vi "AlGaInPAs_v22.vi"(2 "Debug Mode":bool, 3 "Elapsed Time(s)":dbl, 4 "State":enum16{"Edit", "Start", "Run", "End", "Idle"}(ring), 5 "Argument List In":string[](array[string])) -> (0 "Status Out":string, 1 "Argument List Out":string[](array[string]))   [LabVIEW 2011]
uses:
  high_level_proc/source_dilution.ctl
  high_level_proc/source_noDilution.ctl
panel:
  in  "Ring":u16(ring)
  out "source array":refnum<vi>[](array[refnum])
  in  "Zn_bubbler":T1={"Dilution"=FALSE, "Calculated"=0, "MFC1 flow"=0.0, "MFC2 flow"=10.0, "MFC3 flow"=100.0, "Main"={"Flow"=0.0, "Prep"=FALSE, "Run"=FALSE, "Active"=FALSE, "Name"="Zn"}} caption="Al" {"Main"."Flow" format="%.2f"; "MFC1 flow" format="%.4f"; "MFC3 flow" format="%.1f"; "MFC2 flow" format="%.2f"; "Calculated" items=["Flow", "MFC1", "MFC2", "MFC3"]}
  in  "Al_bubbler":T2={"Flow"=0.0, "Prep"=FALSE, "Run"=FALSE, "Active"=FALSE, "Name"="Al"} caption="Al" {"Flow" format="%.2f"}
  in  "Se_bubbler":T1={"Dilution"=FALSE, "Calculated"=0, "MFC1 flow"=0.0, "MFC2 flow"=10.0, "MFC3 flow"=100.0, "Main"={"Flow"=0.0, "Prep"=FALSE, "Run"=FALSE, "Active"=FALSE, "Name"="Se"}} caption="Al" {"Main"."Flow" format="%.2f"; "MFC1 flow" format="%.4f"; "MFC3 flow" format="%.1f"; "MFC2 flow" format="%.2f"; "Calculated" items=["Flow", "MFC1", "MFC2", "MFC3"]}
  in  "P_bubbler":T2={"Flow"=0.0, "Prep"=FALSE, "Run"=FALSE, "Active"=FALSE, "Name"="P liq"} caption="Al" {"Flow" format="%.2f"}
  in  "As_gas":T2={"Flow"=0.0, "Prep"=FALSE, "Run"=FALSE, "Active"=FALSE, "Name"="As gas"} caption="Al" {"Flow" format="%.2f"}
  in  "P_gas":T2={"Flow"=0.0, "Prep"=FALSE, "Run"=FALSE, "Active"=FALSE, "Name"="P gas"} caption="Al" {"Flow" format="%.2f"}
  in  "In_bubbler":T2={"Flow"=0.0, "Prep"=FALSE, "Run"=FALSE, "Active"=FALSE, "Name"="In"} caption="Al" {"Flow" format="%.2f"}
  in  "Ga_bubbler":T1={"Dilution"=FALSE, "Calculated"=0, "MFC1 flow"=0.0, "MFC2 flow"=10.0, "MFC3 flow"=100.0, "Main"={"Flow"=0.0, "Prep"=FALSE, "Run"=FALSE, "Active"=FALSE, "Name"="Ga"}} caption="Al" {"Main"."Flow" format="%.2f"; "MFC1 flow" format="%.4f"; "MFC3 flow" format="%.1f"; "MFC2 flow" format="%.2f"; "Calculated" items=["Flow", "MFC1", "MFC2", "MFC3"]}
  out "prep_done":bool
  out "run started":bool
  out "first":bool=TRUE
  out "is OK?":bool
  in  "prep_time":dbl
  in  "Cancel":bool
  in  "OK":bool
  # "s"
  # "Add pre-run time to run time in editor."
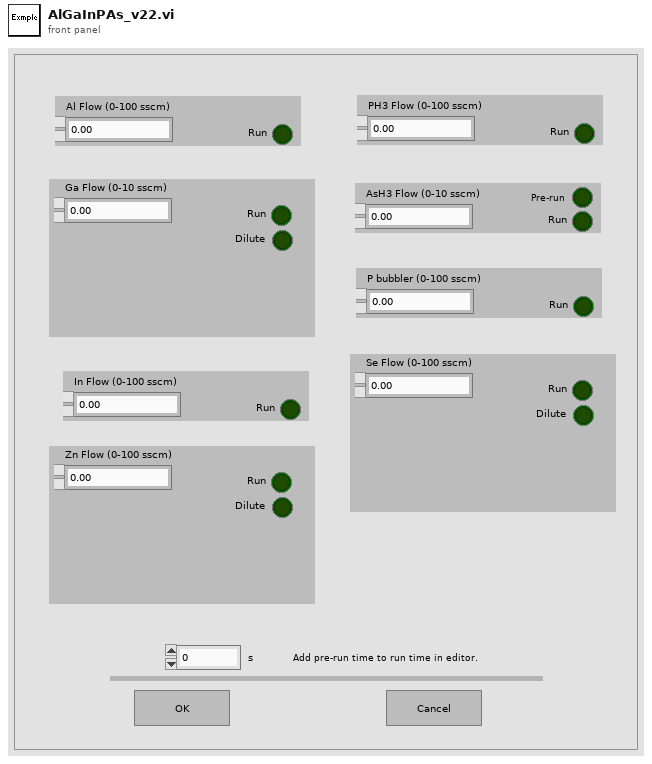
[diagram p1: front panel]
types:
  T1 = typedef "source_dilution.ctl" = cluster{"Dilution":bool, "Calculated":u16, "MFC1 flow":dbl, "MFC2 flow":dbl, "MFC3 flow":dbl, "Main":T2}
  T2 = typedef "source_noDilution.ctl" = cluster{"Flow":dbl, "Prep":bool, "Run":bool, "Active":bool, "Name":string}
  T3 = enum32{"Invalid", "Default", "Floating", "Floating/Auto-Hide", "Modal"}
  T4 = enum16{"Discrete", "Continuous", "Instantaneous", "Finite"}
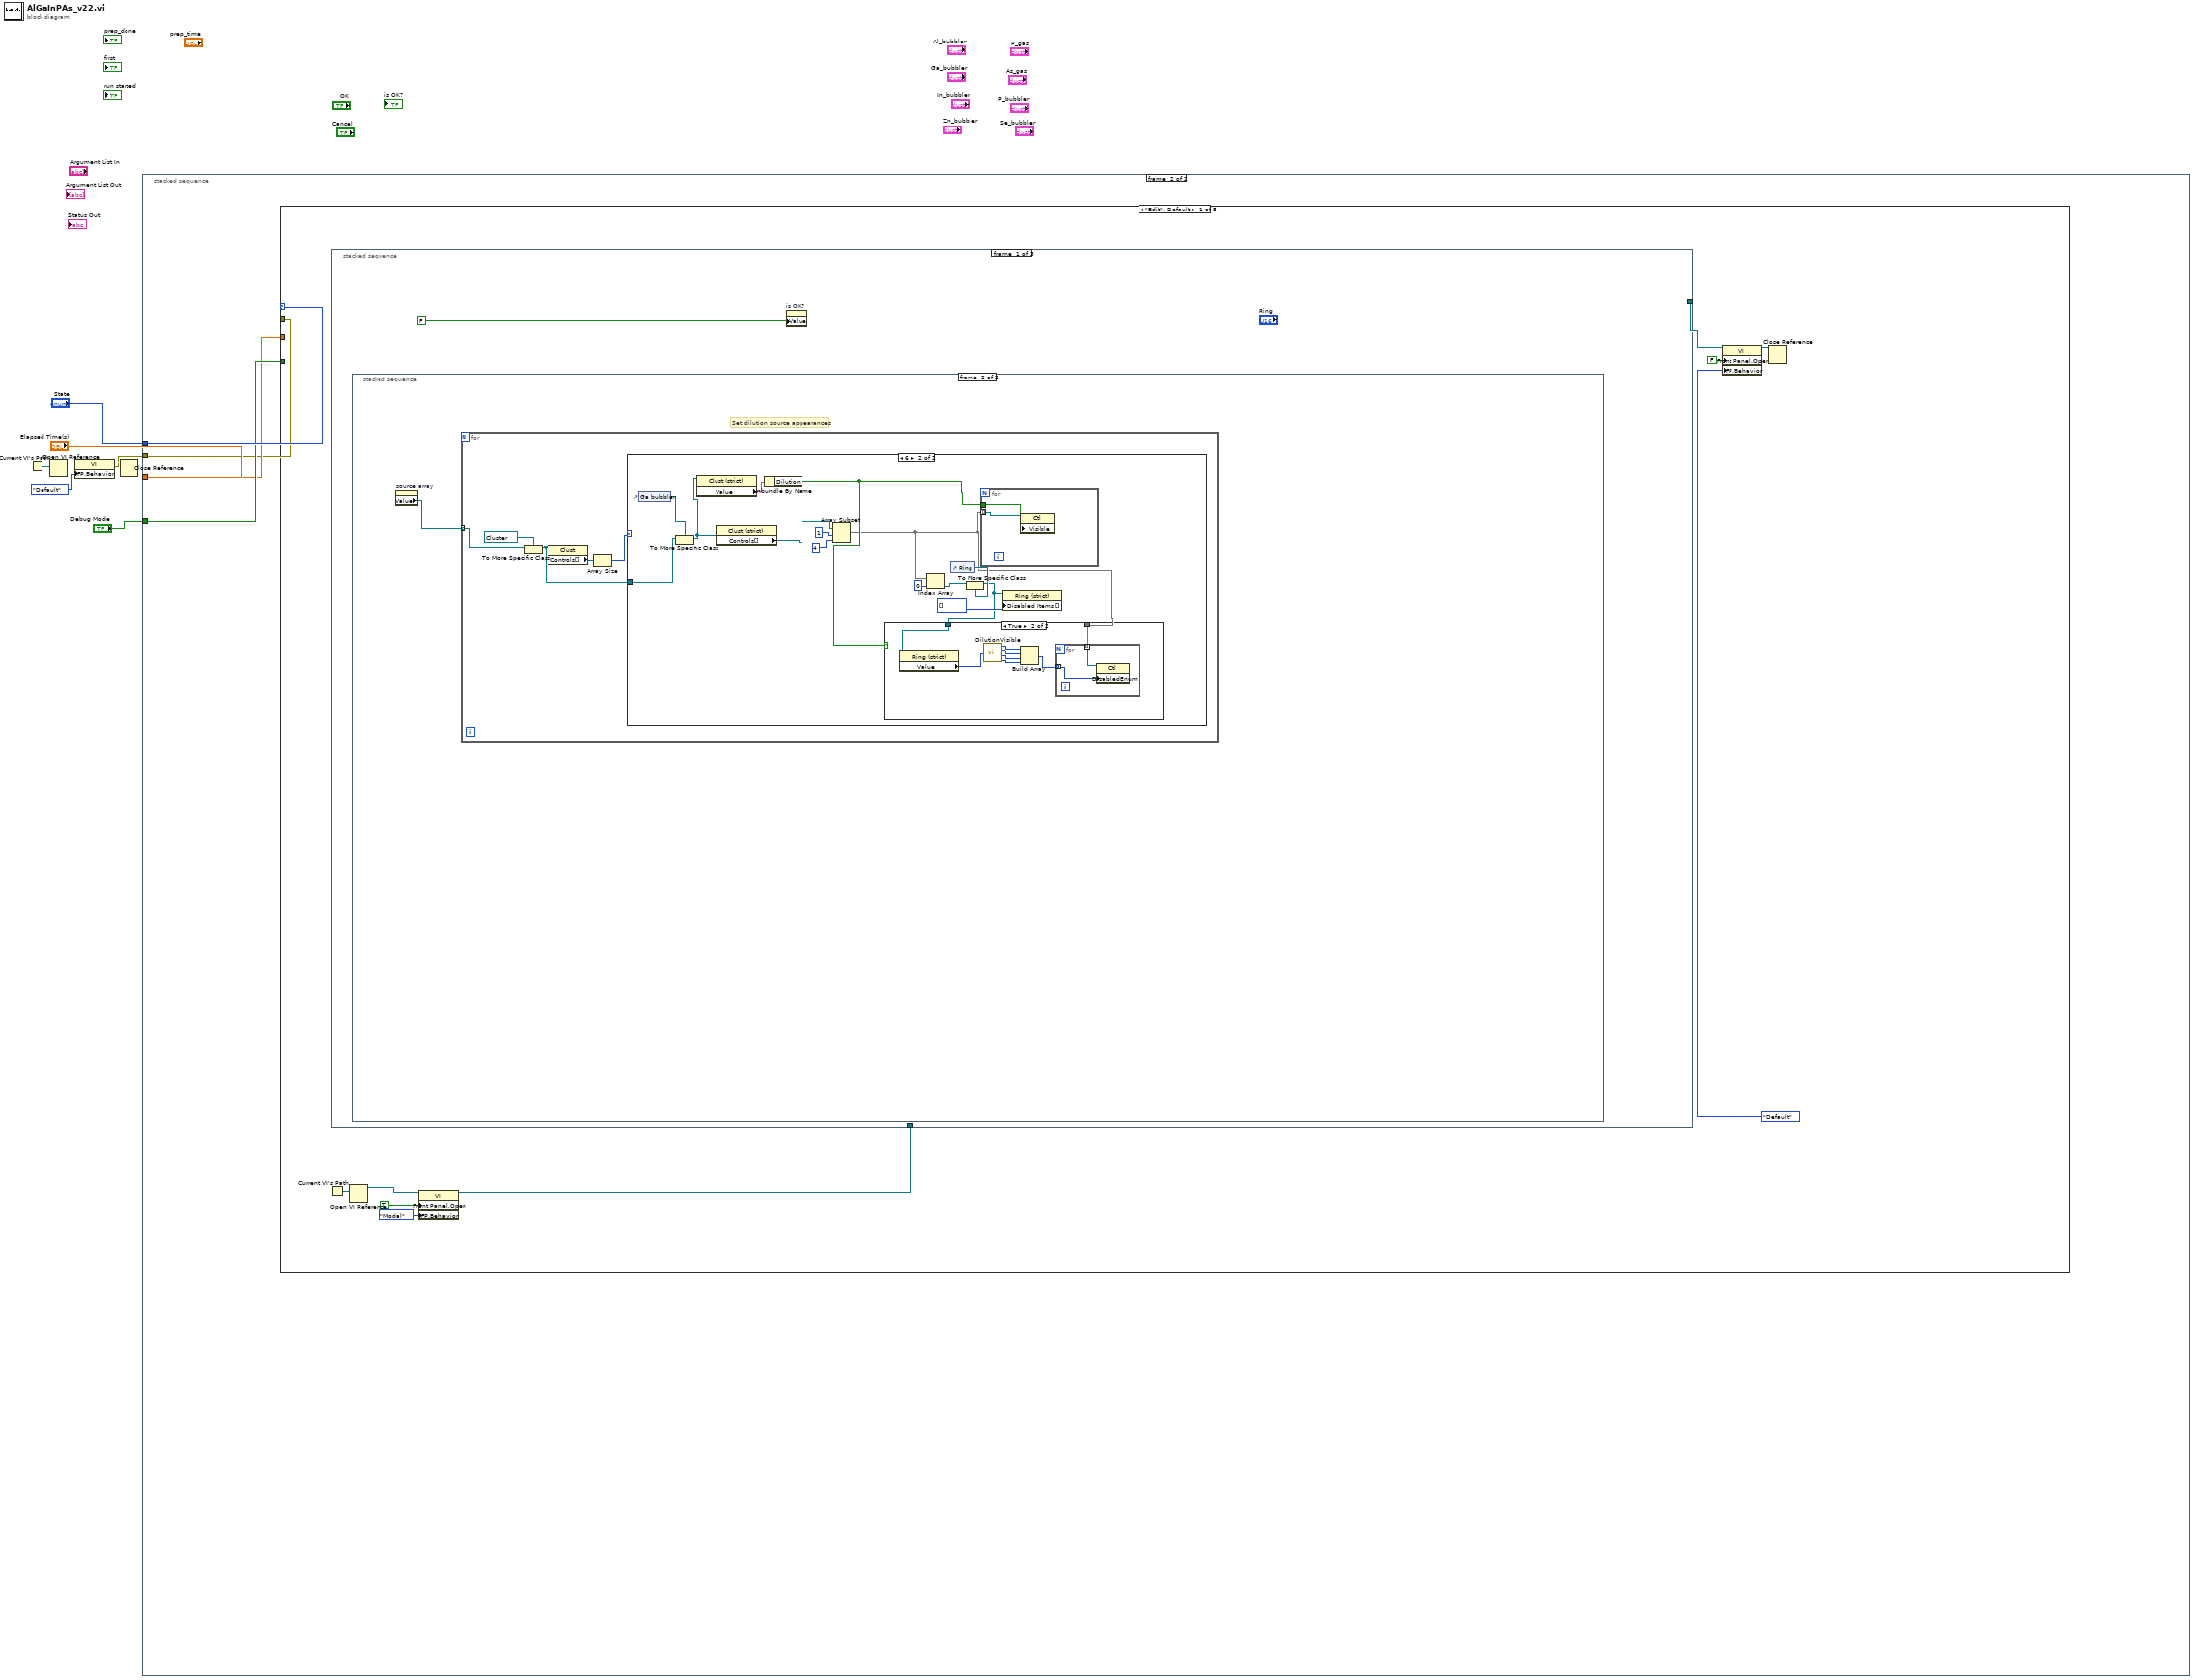
[diagram p0: block diagram]
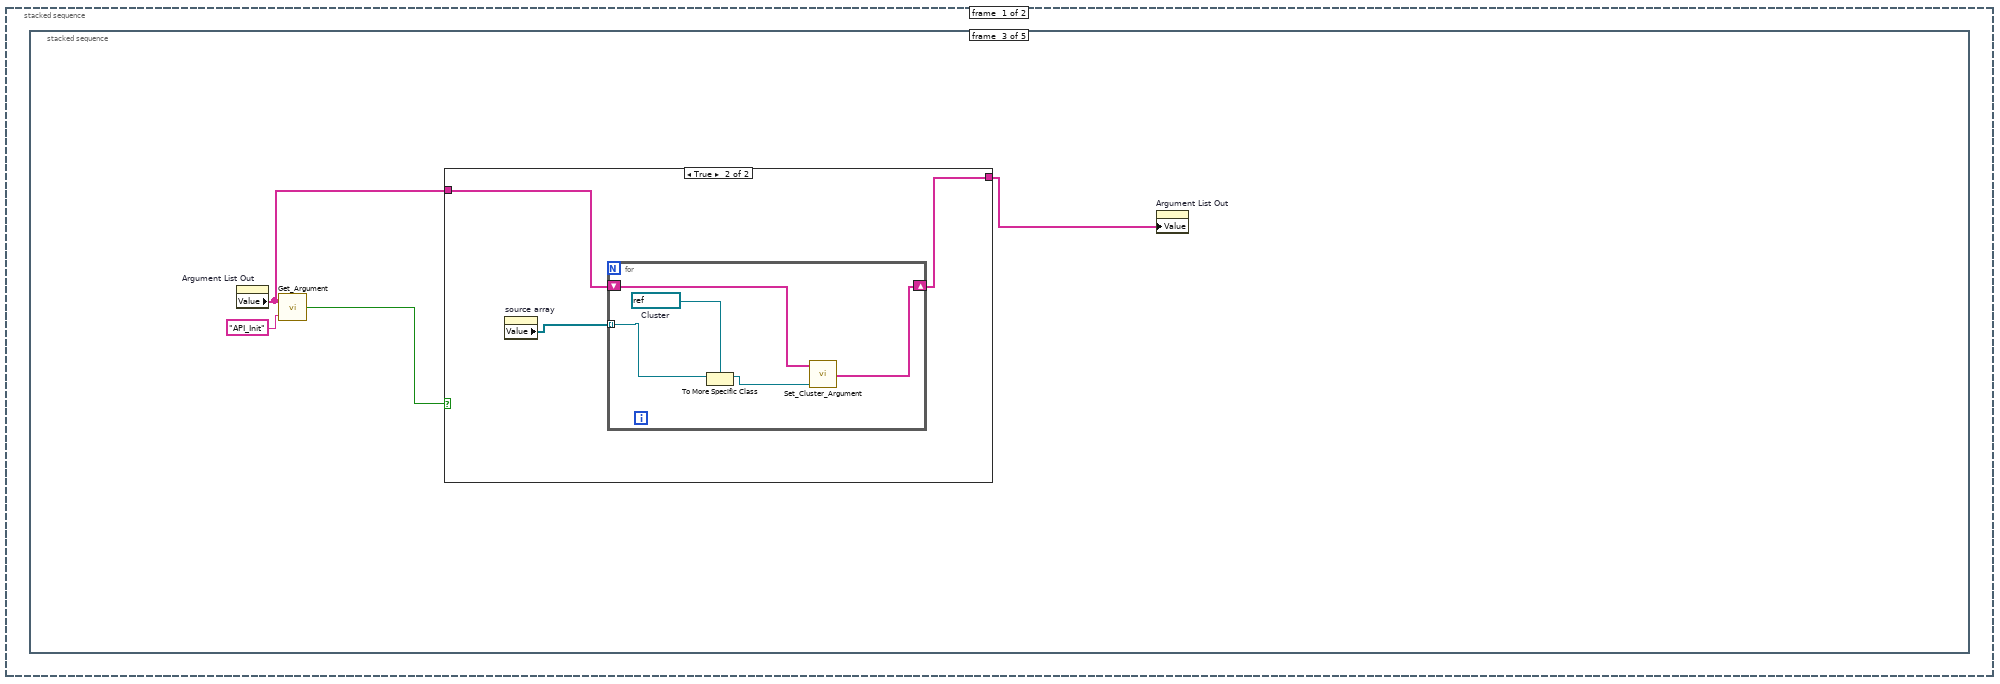
[diagram p2: hidden frame]
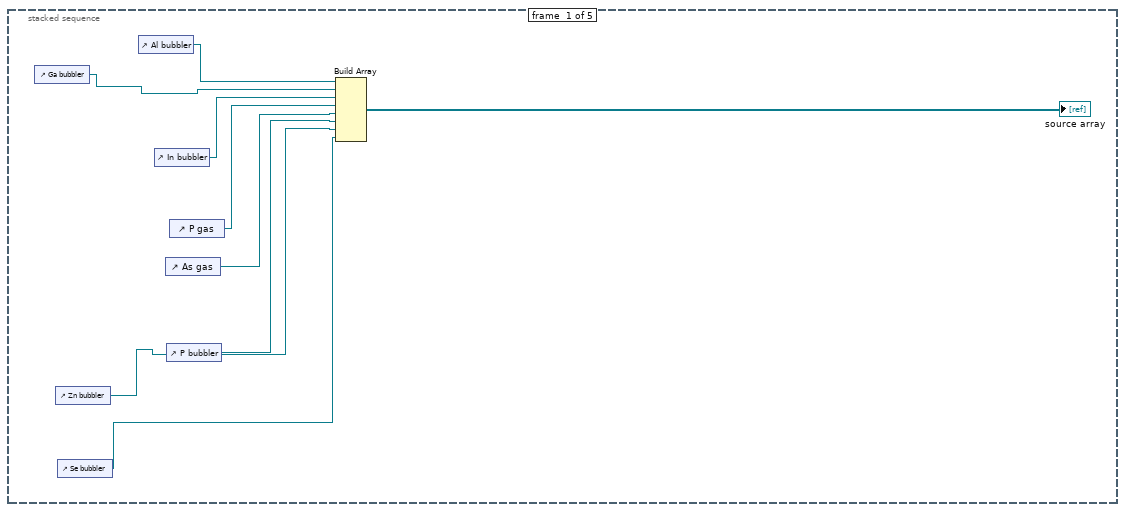
[diagram p3: hidden frame]
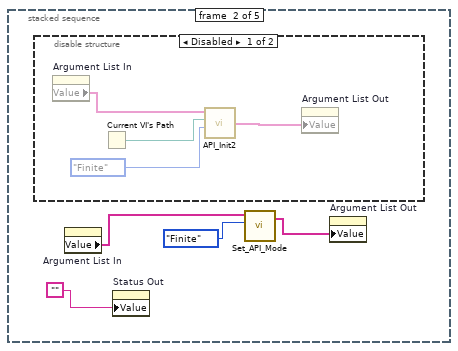
[diagram p4: hidden frame]
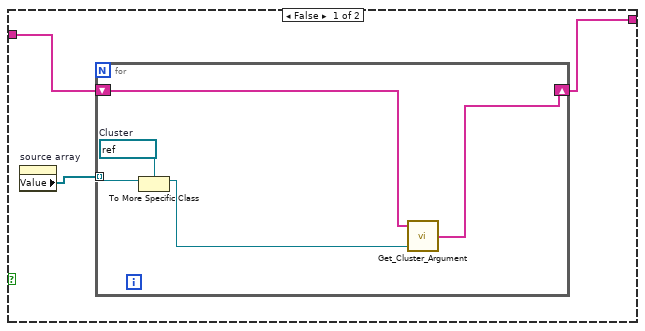
[diagram p6: hidden frame]
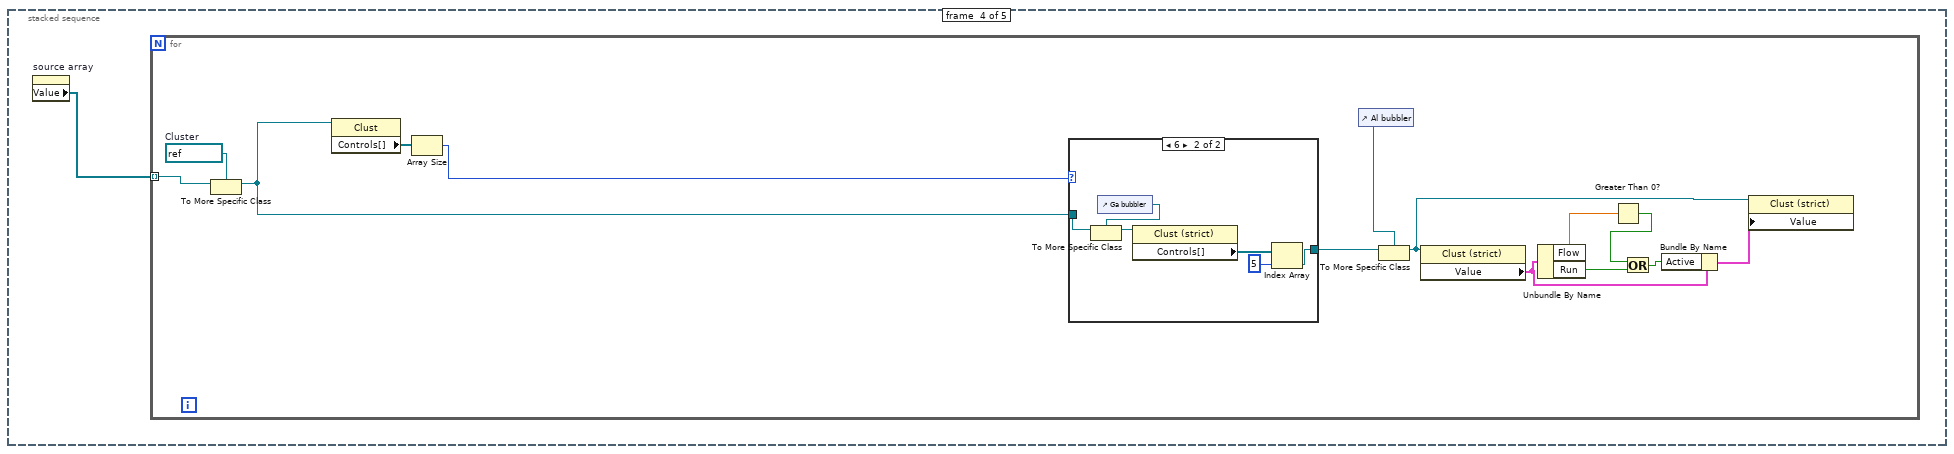
[diagram p7: hidden frame]
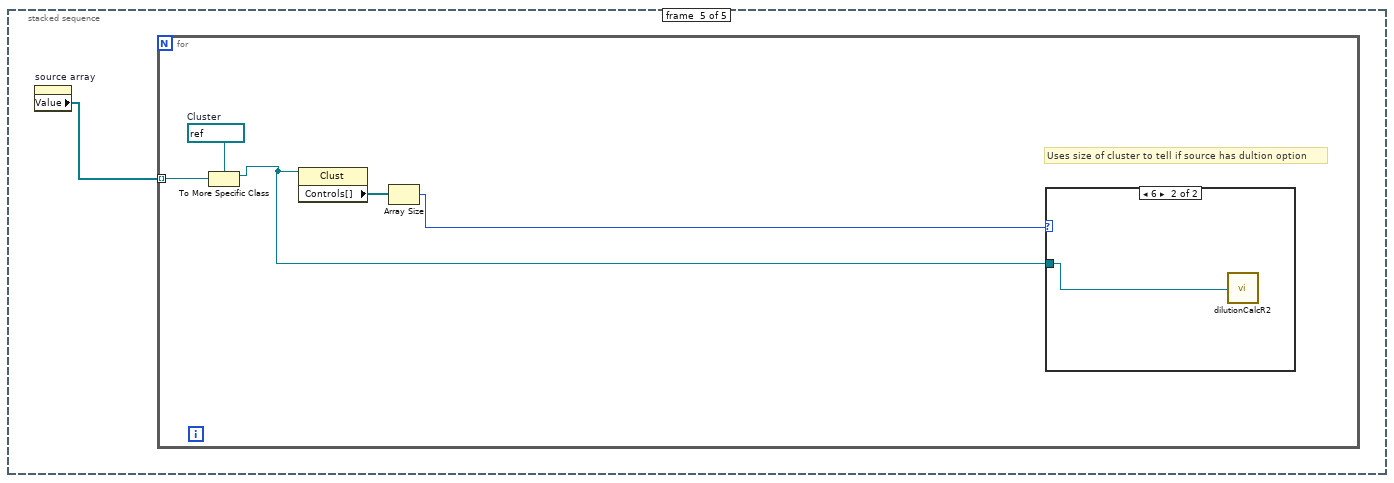
[diagram p9: hidden frame]
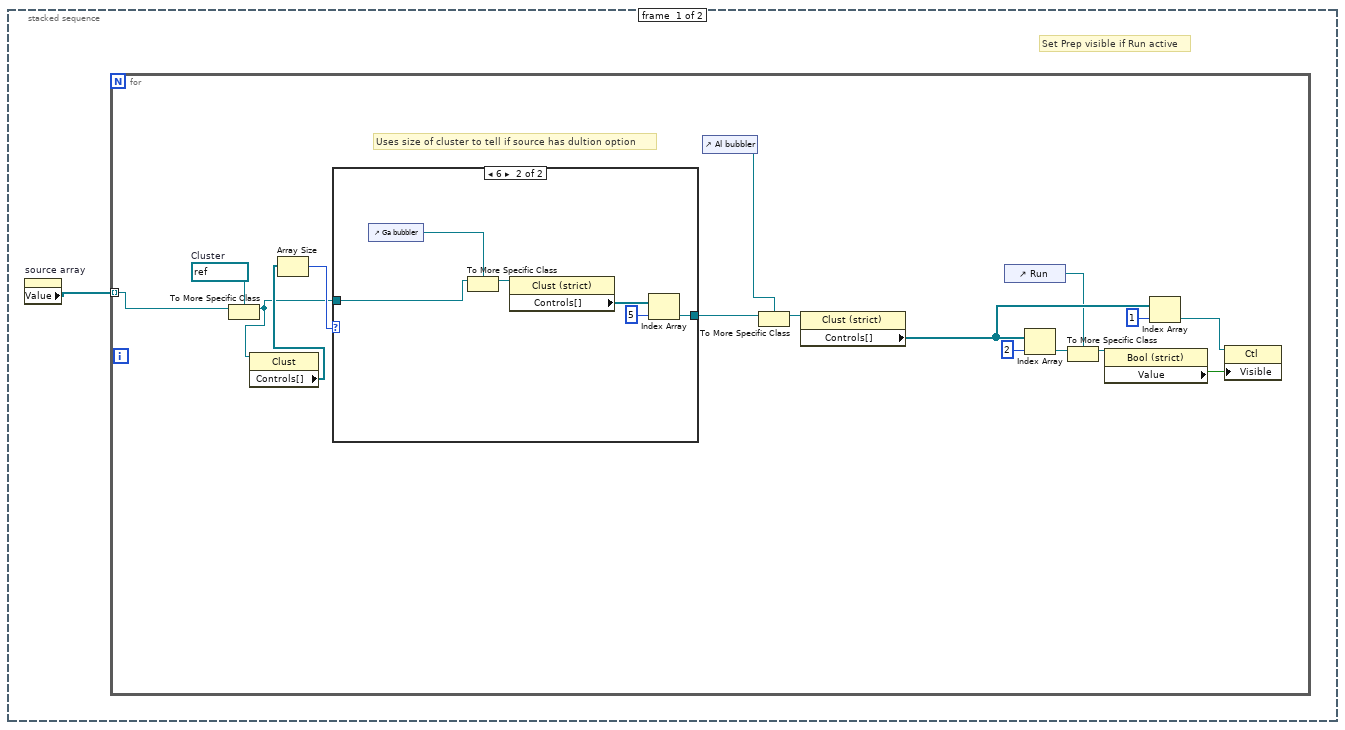
[diagram p11: hidden frame]
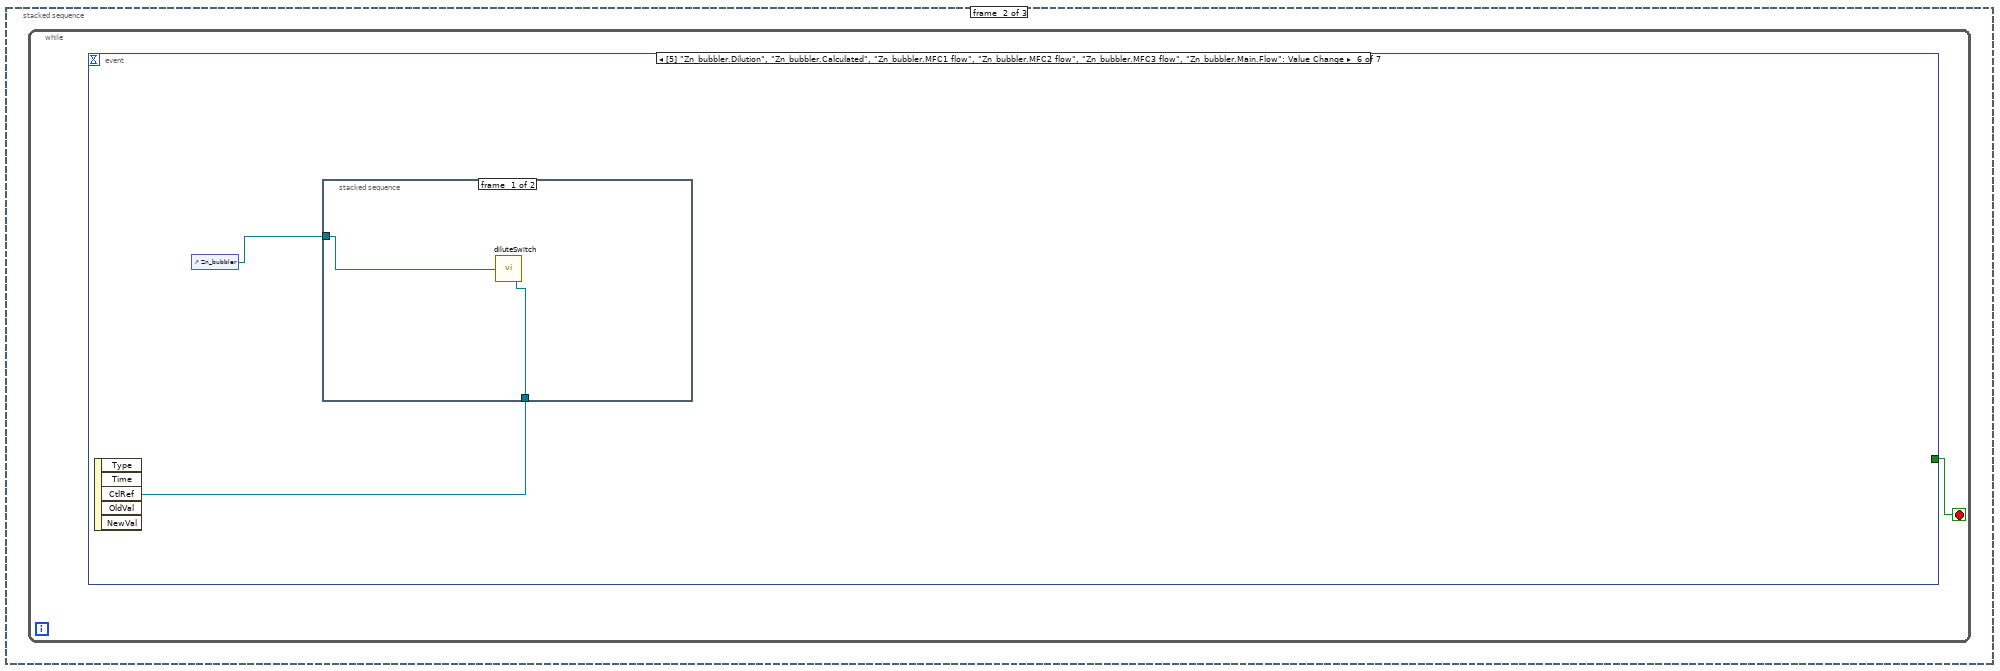
[diagram p15: hidden frame]
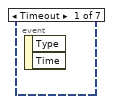
[diagram p16: hidden frame]
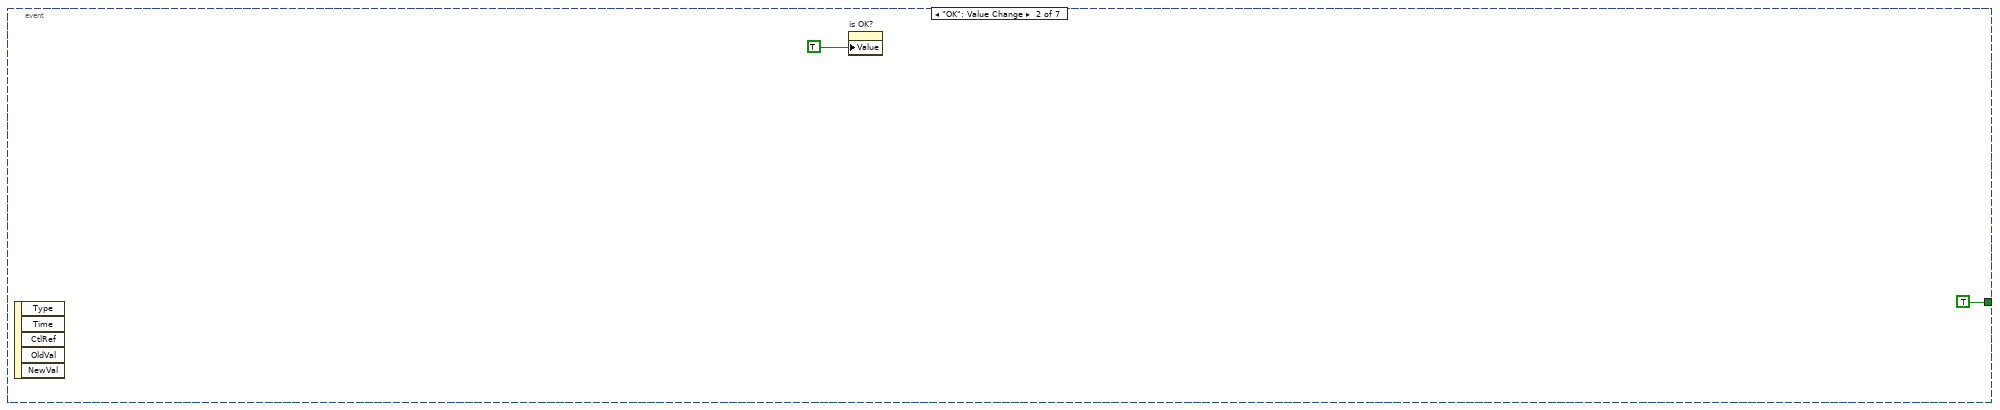
[diagram p17: hidden frame]
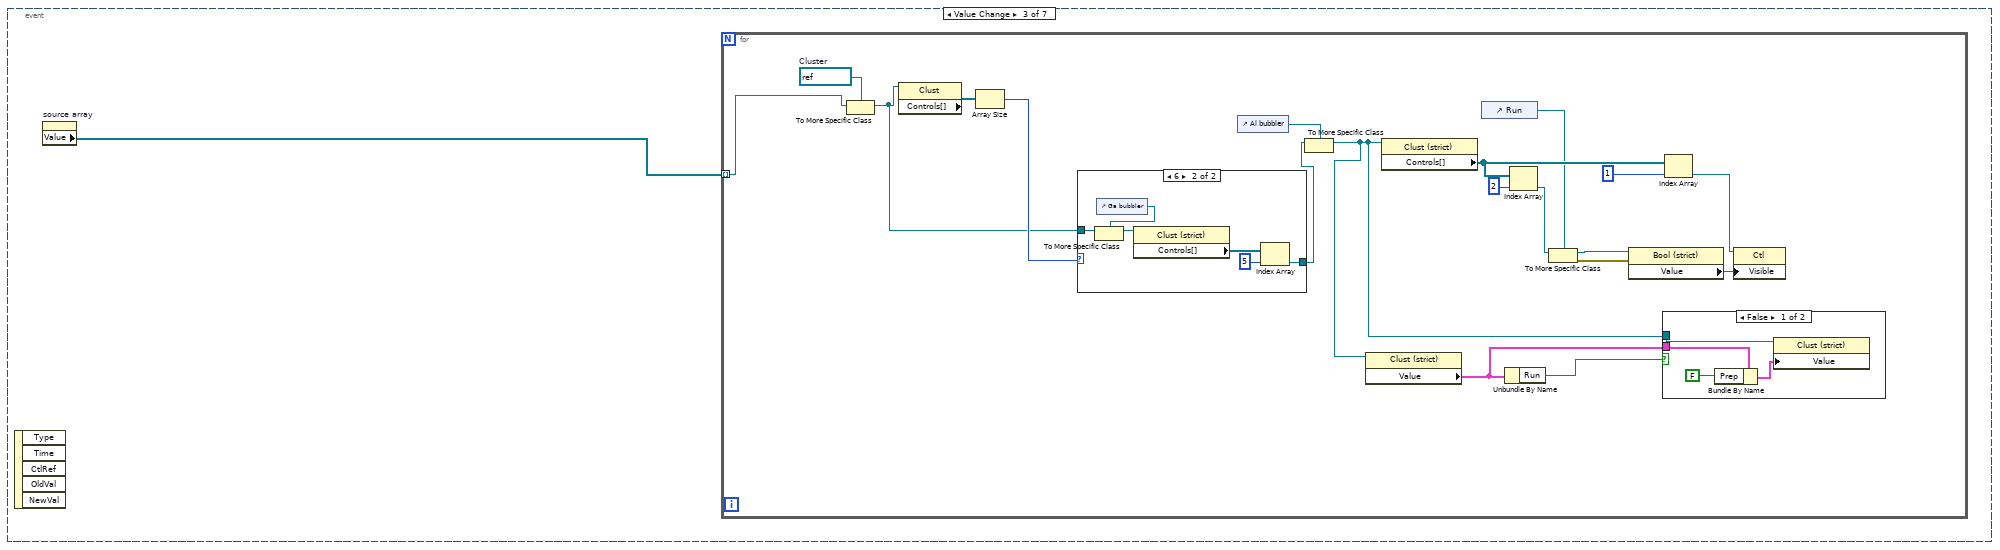
[diagram p18: hidden frame]
diagram:
  n1 = Current VI's Path() -> (path=w5:path)
  n2 = Open VI Reference(vi path=w5) -> (vi reference=w4:refnum<vi>)  [unwired: 1 in, 5 out]
  n3 = property class="VI"(reference=w4, "FP.Behavior"=T3."Default" ("Front Panel Window:Behavior")) -> (reference out=w2:refnum<vi>, error out=w1:errorcluster)  [unwired: 1 in]
  n4 = Close Reference(reference=w2) -> ()  [unwired: 1 in, 1 out]
  n5 = stacked-sequence {
    tunnel: "State" -> [_ w78]
    tunnel: "Debug Mode" -> [_ w77]
    tunnel: "Elapsed Time(s)" -> [_ w76]
    tunnel: w1 -> [_ w75]
    frame #0 {
      n6 = stacked-sequence {
        frame #0 {
          n7 = control-ref of="Ga bubbler"() -> (w12:refnum<vi>)
          n8 = control-ref of="Zn bubbler"() -> (w11:refnum<vi>)
          n9 = control-ref of="Se bubbler"() -> (w10:refnum<vi>)
          n10 = control-ref of="Al bubbler"() -> (w17:refnum<vi>)
          n11 = control-ref of="In bubbler"() -> (w16:refnum<vi>)
          n12 = control-ref of="As gas"() -> (w14:refnum<vi>)
          n13 = control-ref of="P bubbler"() -> (w13:refnum<vi>)
          n14 = control-ref of="P gas"() -> (w15:refnum<vi>)
          n15 = Build Array(w17, w12, w16, w15, w14, w13, w11, w10) -> (→"source array":refnum<vi>[])
        }
        frame #1 {
          n16 = disable-structure shown="Disabled" {
            frame Disabled {
              n17 = property on="Argument List In" class="Arr (strict)"() -> ("Value"=w25:string[])  [unwired: 2 in, 2 out]
              n18 = Current VI's Path() -> (path=w22:path)
              n19 = call "API_Init2.vi"("API Mode"=T4."Finite", "VI Path"=w22, "Argument List In"=w25) -> ("Argument List Out"=w24:string[])  [unwired: 1 in]
              n20 = property on="Argument List Out" class="Arr (strict)"("Value"=w24) -> ()  [unwired: 2 in, 2 out]
            }
            frame Enabled {
            }
          }
          n21 = property on="Argument List In" class="Arr (strict)"() -> ("Value"=w20:string[])  [unwired: 2 in, 2 out]
          n22 = property on="Status Out" class="Str"("Value"="") -> ()  [unwired: 2 in, 2 out]
          n23 = call "Set_API_Mode.vi"("API Mode"=T4."Finite", "Argument List In"=w20) -> ("Argument List Out"=w18:string[])  [unwired: 3 in]
          n24 = property on="Argument List Out" class="Arr (strict)"("Value"=w18) -> ()  [unwired: 2 in, 2 out]
        }
        frame #2 {
          n25 = property on="Argument List Out" class="Arr (strict)"() -> ("Value"=w27:string[])  [unwired: 2 in, 2 out]
          n26 = call "Get_Argument.vi"("Argument"="API_Init", "Argument List"=w27) -> ("Enabled"=w28:bool)
          n27 = case shown="True" w28 {
            tunnel: w27 -> [w32 w40]
            tunnel: [w30 w39] -> w26
            frame False {
              n28 = property on="source array" class="Arr (strict)"() -> ("Value"=w31:refnum<vi>[])  [unwired: 2 in, 2 out]
              n29 = for {
                shift-right: [w36] -> w30
                shift-left: w32 -> [w37]
                tunnel: w31 -> [w35] mode=indexing
                w33 = refnum<vi> refnum  # Cluster
                n30 = To More Specific Class(target class=w33, reference=w35) -> (specific class reference=w34:refnum<vi>)  [unwired: 1 in, 1 out]
                n31 = call "Get_Cluster_Argument.vi"("source"=w34, "Argument List In"=w37) -> ("Argument List Out"=w36:string[])  [unwired: 1 in]
              }
            }
            frame True {
              n32 = property on="source array" class="Arr (strict)"() -> ("Value"=w38:refnum<vi>[])  [unwired: 2 in, 2 out]
              n33 = for {
                shift-right: [w44] -> w39
                shift-left: w40 -> [w45]
                tunnel: w38 -> [w43] mode=indexing
                w42 = refnum<vi> refnum  # Cluster
                n34 = To More Specific Class(target class=w42, reference=w43) -> (specific class reference=w41:refnum<vi>)  [unwired: 1 in, 1 out]
                n35 = call "Set_Cluster_Argument.vi"("Clust Refnum"=w41, "Argument List In"=w45) -> ("Argument List Out"=w44:string[])  [unwired: 1 in]
              }
            }
          }
          n36 = property on="Argument List Out" class="Arr (strict)"("Value"=w26) -> ()  [unwired: 2 in, 2 out]
        }
        frame #3 {
          n37 = property on="source array" class="Arr (strict)"() -> ("Value"=w46:refnum<vi>[])  [unwired: 2 in, 2 out]
          n38 = for {
            tunnel: w46 -> [w49] mode=indexing
            w47 = refnum<vi> refnum  # Cluster
            n39 = To More Specific Class(target class=w47, reference=w49) -> (specific class reference=w48:refnum<vi>)  [unwired: 1 in, 1 out]
            n40 = property class="Clust"(reference=w48) -> ("Controls[]"=w51:refnum<vi>[])  [unwired: 1 in, 2 out]
            n41 = Array Size(array=w51) -> (size(s)=w52:i32)
            n42 = case shown="6" w52 {
              tunnel: [w61 w63] -> w50
              tunnel: w48 -> [w61 w66]
              frame Default {
              }
              frame 6 {
                n43 = control-ref of="Ga bubbler"() -> (w62:refnum<vi>)
                n44 = To More Specific Class(target class=w62, reference=w66) -> (specific class reference=w65:refnum<vi>)  [unwired: 1 in, 1 out]
                n45 = property class="Clust (strict)"(reference=w65) -> ("Controls[]"=w64:refnum<vi>[])  [unwired: 1 in, 2 out]
                n46 = Index Array(array=w64, index=5) -> (element=w63:refnum<vi>)
              }
            }
            n47 = control-ref of="Al bubbler"() -> (w54:refnum<vi>)
            n48 = To More Specific Class(target class=w54, reference=w50) -> (specific class reference=w53:refnum<vi>)  [unwired: 1 in, 1 out]
            n49 = property class="Clust (strict)"(reference=w53) -> ("Value"=w57:T2)  [unwired: 1 in, 2 out]
            n50 = Unbundle By Name(w57) -> ("Flow"=w60:dbl, "Run"=w58:bool)
            n51 = Greater Than 0?(x=w60) -> (x > 0?=w59:bool)
            n52 = Or(x=w59, y=w58) -> (x .or. y?=w55:bool)
            n53 = Bundle By Name(cluster=w57, "Active"=w55) -> (w56:T2)
            n54 = property class="Clust (strict)"(reference=w53, "Value"=w56) -> ()  [unwired: 1 in, 2 out]
          }
        }
        frame #4 {
          n55 = property on="source array" class="Arr (strict)"() -> ("Value"=w68:refnum<vi>[])  [unwired: 2 in, 2 out]
          n56 = for {
            tunnel: w68 -> [w72] mode=indexing
            w70 = refnum<vi> refnum  # Cluster
            # "Uses size of cluster to tell if source has dultion option"
            n57 = To More Specific Class(target class=w70, reference=w72) -> (specific class reference=w71:refnum<vi>)  [unwired: 1 in, 1 out]
            n58 = property class="Clust"(reference=w71) -> ("Controls[]"=w69:refnum<vi>[])  [unwired: 1 in, 2 out]
            n59 = Array Size(array=w69) -> (size(s)=w73:i32)
            n60 = case shown="6" w73 {
              tunnel: w71 -> [_ w74]
              frame Default {
              }
              frame 6 {
                n61 = call "dilutionCalcR2.vi"("Clust Refnum"=w74) -> ()
              }
            }
          }
        }
      }
    }
    frame #1 {
      n62 = case shown="\"Edit\", Default" w78 {
        tunnel: w77 -> [_ w214 w230 _ _]
        tunnel: w76 -> [_ _ w231 _ _]
        tunnel: w75 -> [_ _ _ _ _]
        frame "Edit", Default {
          n63 = Current VI's Path() -> (path=w83:path)
          n64 = Open VI Reference(vi path=w83) -> (vi reference=w82:refnum<vi>)  [unwired: 1 in, 5 out]
          n65 = property class="VI"(reference=w82, "Front Panel.Open"=TRUE ("Front Panel Window:Open"), "FP.Behavior"=T3."Modal" ("Front Panel Window:Behavior")) -> (reference out=w80:refnum<vi>)  [unwired: 1 in, 1 out]
          n66 = stacked-sequence {
            tunnel: [_ _ w197] -> w85
            tunnel: w80 -> [_ _ w197]
            frame #0 {
              n67 = stacked-sequence {
                frame #0 {
                  # "Set Prep visible if Run active"
                  n68 = property on="source array" class="Arr (strict)"() -> ("Value"=w89:refnum<vi>[])  [unwired: 2 in, 2 out]
                  n69 = for {
                    tunnel: w89 -> [w94] mode=indexing
                    w93 = refnum<vi> refnum  # Cluster
                    # "Uses size of cluster to tell if source has dultion option"
                    n70 = To More Specific Class(target class=w93, reference=w94) -> (specific class reference=w90:refnum<vi>)  [unwired: 1 in, 1 out]
                    n71 = property class="Clust"(reference=w90) -> ("Controls[]"=w92:refnum<vi>[])  [unwired: 1 in, 2 out]
                    n72 = Array Size(array=w92) -> (size(s)=w91:i32)
                    n73 = case shown="6" w91 {
                      tunnel: w90 -> [w106 w109]
                      tunnel: [w106 w110] -> w96
                      frame Default {
                      }
                      frame 6 {
                        n74 = control-ref of="Ga bubbler"() -> (w107:refnum<vi>)
                        n75 = To More Specific Class(target class=w107, reference=w109) -> (specific class reference=w108:refnum<vi>)  [unwired: 1 in, 1 out]
                        n76 = property class="Clust (strict)"(reference=w108) -> ("Controls[]"=w112:refnum<vi>[])  [unwired: 1 in, 2 out]
                        n77 = Index Array(array=w112, index=5) -> (element=w110:refnum<vi>)
                      }
                    }
                    n78 = control-ref of="Al bubbler"() -> (w97:refnum<vi>)
                    n79 = To More Specific Class(target class=w97, reference=w96) -> (specific class reference=w103:refnum<vi>)  [unwired: 1 in, 1 out]
                    n80 = property class="Clust (strict)"(reference=w103) -> ("Controls[]"=w102:refnum<vi>[])  [unwired: 1 in, 2 out]
                    n81 = control-ref of="Run"() -> (w95:refnum<vi>)
                    n82 = Index Array(array=w102, index=2) -> (element=w100:refnum<vi>)
                    n83 = To More Specific Class(target class=w95, reference=w100) -> (specific class reference=w99:refnum<vi>)  [unwired: 1 in, 1 out]
                    n84 = property class="Bool (strict)"(reference=w99) -> ("Value"=w98:bool)  [unwired: 1 in, 2 out]
                    n85 = Index Array(array=w102, index=1) -> (element=w104:refnum<vi>)
                    n86 = property class="Ctl"(reference=w104, "Visible"=w98) -> ()  [unwired: 1 in, 2 out]
                  }
                }
                frame #1 {
                  # "Set dilution source appearances"
                  n87 = property on="source array" class="Arr (strict)"() -> ("Value"=w113:refnum<vi>[])  [unwired: 2 in, 2 out]
                  n88 = for {
                    tunnel: w113 -> [w118] mode=indexing
                    n89 = To More Specific Class(target class=refnum<vi> refnum, reference=w118) -> (specific class reference=w114:refnum<vi>)  [unwired: 1 in, 1 out]
                    n90 = property class="Clust"(reference=w114) -> ("Controls[]"=w116:refnum<vi>[])  [unwired: 1 in, 2 out]
                    n91 = Array Size(array=w116) -> (size(s)=w115:i32)
                    n92 = case shown="6" w115 {
                      tunnel: w114 -> [_ w132]
                      frame Default {
                      }
                      frame 6 {
                        n93 = control-ref of="Ga bubbler"() -> (w131:refnum<vi>)
                        n94 = To More Specific Class(target class=w131, reference=w132) -> (specific class reference=w129:refnum<vi>)  [unwired: 1 in, 1 out]
                        n95 = property class="Clust (strict)"(reference=w129) -> ("Value"=w130:T1)  [unwired: 1 in, 2 out]
                        n96 = property class="Clust (strict)"(reference=w129) -> ("Controls[]"=w128:refnum<vi>[])  [unwired: 1 in, 2 out]
                        n97 = Unbundle By Name(w130) -> ("Dilution"=w122:bool)
                        n98 = Array Subset(array=w128, index=1, length=4) -> (w119:refnum<vi>[])
                        n99 = Index Array(array=w119, index=0) -> (element=w121:refnum<vi>)
                        n100 = control-ref of="Ring"() -> (w124:refnum<vi>)
                        n101 = To More Specific Class(target class=w124, reference=w121) -> (specific class reference=w120:refnum<vi>)  [unwired: 1 in, 1 out]
                        n102 = case shown="True" w122 {
                          tunnel: w120 -> [_ w140]
                          tunnel: w119 -> [_ w133]
                          frame False {
                          }
                          frame True {
                            n103 = property class="Ring (strict)"(reference=w140) -> ("Value"=w139:u16)  [unwired: 1 in, 2 out]
                            n104 = call "DilutionVisible.vi"("calculated"=w139) -> ("flow"=w138:u16, "MFC1"=w137:u16, "MFC2"=w136:u16, "MFC3"=w135:u16)
                            n105 = Build Array(w138, w137, w136, w135) -> (w134:u16[])
                            n106 = for {
                              tunnel: w134 -> [w141] mode=indexing
                              tunnel: w133 -> [w142] mode=indexing
                              n107 = property class="Ctl"(reference=w142, "DisabledEnum"=w141) -> ()  [unwired: 1 in, 2 out]
                            }
                          }
                        }
                        n108 = for {
                          tunnel: w119 -> [w144] mode=indexing
                          tunnel: w122 -> [w143]
                          n109 = property class="Ctl"(reference=w144, "Visible"=w143) -> ()  [unwired: 1 in, 2 out]
                        }
                        n110 = property class="Ring (strict)"(reference=w120, "Disabled Items []"=i32[] []) -> ()  [unwired: 1 in, 2 out]
                      }
                    }
                  }
                }
              }
              n111 = property on="is OK?" class="Bool (strict)"("Value"=FALSE ("is OK?")) -> ()  [unwired: 2 in, 2 out]
            }
            frame #1 {
              n112 = while {
                stop <- w145 stop-if-true
                n113 = event shown="[5] \"Zn_bubbler.Dilution\", \"Zn_bubbler.Calculated\", \"Zn_bubbler.MFC1 flow\", \"Zn_bubbler.MFC2 flow\", \"Zn_bubbler.MFC3 flow\", \"Zn_bubbler.Main.Flow\": Value Change" {
                  selector: _ -> [_ _ _ _ _ _ _]
                  dyn-events: _ -> [_ _ _ _ _ _ _]
                  timeout: _ -> [_ _ _ _ _ _ _]
                  tunnel: [_ TRUE _ TRUE _ _ _] -> w145
                  event Timeout {
                    n114 = event-data() -> ()  [unwired: 1 in, 2 out]
                  }
                  event "OK": Value Change {
                    n115 = event-data() -> ()  [unwired: 1 in, 5 out]
                    n116 = property on="is OK?" class="Bool (strict)"("Value"=TRUE ("is OK?")) -> ()  [unwired: 2 in, 2 out]
                  }
                  event Value Change {
                    n117 = event-data() -> ()  [unwired: 1 in, 5 out]
                    n118 = property on="source array" class="Arr (strict)"() -> ("Value"=w148:refnum<vi>[])  [unwired: 2 in, 2 out]
                    n119 = for {
                      tunnel: w148 -> [w151] mode=indexing
                      w149 = refnum<vi> refnum  # Cluster
                      n120 = To More Specific Class(target class=w149, reference=w151) -> (specific class reference=w150:refnum<vi>)  [unwired: 1 in, 1 out]
                      n121 = property class="Clust"(reference=w150) -> ("Controls[]"=w153:refnum<vi>[])  [unwired: 1 in, 2 out]
                      n122 = Array Size(array=w153) -> (size(s)=w152:i32)
                      n123 = case shown="6" w152 {
                        tunnel: w150 -> [w168 w171]
                        tunnel: [w168 w172] -> w155
                        frame Default {
                        }
                        frame 6 {
                          n124 = control-ref of="Ga bubbler"() -> (w169:refnum<vi>)
                          n125 = To More Specific Class(target class=w169, reference=w171) -> (specific class reference=w170:refnum<vi>)  [unwired: 1 in, 1 out]
                          n126 = property class="Clust (strict)"(reference=w170) -> ("Controls[]"=w174:refnum<vi>[])  [unwired: 1 in, 2 out]
                          n127 = Index Array(array=w174, index=5) -> (element=w172:refnum<vi>)
                        }
                      }
                      n128 = control-ref of="Al bubbler"() -> (w159:refnum<vi>)
                      n129 = To More Specific Class(target class=w159, reference=w155) -> (specific class reference=w156:refnum<vi>)  [unwired: 1 in, 1 out]
                      n130 = property class="Clust (strict)"(reference=w156) -> ("Value"=w158:T2)  [unwired: 1 in, 2 out]
                      n131 = property class="Clust (strict)"(reference=w156) -> ("Controls[]"=w165:refnum<vi>[])  [unwired: 1 in, 2 out]
                      n132 = control-ref of="Run"() -> (w154:refnum<vi>)
                      n133 = Unbundle By Name(w158) -> ("Run"=w157:bool)
                      n134 = Index Array(array=w165, index=2) -> (element=w163:refnum<vi>)
                      n135 = To More Specific Class(target class=w154, reference=w163) -> (specific class reference=w162:refnum<vi>, error out=w161:errorcluster)  [unwired: 1 in]
                      n136 = property class="Bool (strict)"(reference=w162, error in=w161) -> ("Value"=w160:bool)  [unwired: 2 out]
                      n137 = case shown="False" w157 {
                        tunnel: w158 -> [w178 _]
                        tunnel: w156 -> [w175 _]
                        frame False {
                          n138 = Bundle By Name(cluster=w178, "Prep"=FALSE) -> (w176:T2)
                          n139 = property class="Clust (strict)"(reference=w175, "Value"=w176) -> ()  [unwired: 1 in, 2 out]
                        }
                        frame True {
                        }
                      }
                      n140 = Index Array(array=w165, index=1) -> (element=w166:refnum<vi>)
                      n141 = property class="Ctl"(reference=w166, "Visible"=w160) -> ()  [unwired: 1 in, 2 out]
                    }
                  }
                  event "Cancel": Value Change {
                    n142 = event-data() -> ()  [unwired: 1 in, 5 out]
                  }
                  event Value Change {
                    n143 = event-data() -> ("CtlRef"=w180:refnum<vi>)  [unwired: 1 in, 4 out]
                    n144 = control-ref of="Ga_bubbler"() -> (w181:refnum<vi>)
                    n145 = stacked-sequence {
                      tunnel: w181 -> [w183 w184]
                      tunnel: w180 -> [w182 _]
                      frame #0 {
                        n146 = call "diluteSwitch.vi"("Ctl Refnum"=w182, "Clust Refnum"=w183) -> ()
                      }
                      frame #1 {
                        n147 = call "dilutionCalcR2.vi"("Clust Refnum"=w184) -> ()
                      }
                    }
                  }
                  event Value Change {
                    n148 = event-data() -> ("CtlRef"=w185:refnum<vi>)  [unwired: 1 in, 4 out]
                    n149 = control-ref of="Zn_bubbler"() -> (w186:refnum<vi>)
                    n150 = stacked-sequence {
                      tunnel: w186 -> [w188 w189]
                      tunnel: w185 -> [w187 _]
                      frame #0 {
                        n151 = call "diluteSwitch.vi"("Ctl Refnum"=w187, "Clust Refnum"=w188) -> ()
                      }
                      frame #1 {
                        n152 = call "dilutionCalcR2.vi"("Clust Refnum"=w189) -> ()
                      }
                    }
                  }
                  event Value Change {
                    n153 = event-data() -> ("CtlRef"=w190:refnum<vi>)  [unwired: 1 in, 4 out]
                    n154 = control-ref of="Se_bubbler"() -> (w191:refnum<vi>)
                    n155 = stacked-sequence {
                      tunnel: w191 -> [w193 w194]
                      tunnel: w190 -> [w192 _]
                      frame #0 {
                        n156 = call "diluteSwitch.vi"("Ctl Refnum"=w192, "Clust Refnum"=w193) -> ()
                      }
                      frame #1 {
                        n157 = call "dilutionCalcR2.vi"("Clust Refnum"=w194) -> ()
                      }
                    }
                  }
                }
              }
            }
            frame #2 {
              n158 = property on="Argument List Out" class="Arr (strict)"() -> ("Value"=w196:string[])  [unwired: 2 in, 2 out]
              n159 = property on="is OK?" class="Bool (strict)"() -> ("Value"=w198:bool)  [unwired: 2 in, 2 out]
              n160 = case shown="True" w198 {
                tunnel: w196 -> [w199 w205]
                tunnel: [w199 w201] -> w195
                frame False {
                }
                frame True {
                  n161 = property on="source array" class="Arr (strict)"() -> ("Value"=w204:refnum<vi>[])  [unwired: 2 in, 2 out]
                  n162 = for {
                    shift-right: [w209] -> w202
                    shift-left: w205 -> [w210]
                    tunnel: w204 -> [w208] mode=indexing
                    w207 = refnum<vi> refnum  # Cluster
                    n163 = To More Specific Class(target class=w207, reference=w208) -> (specific class reference=w206:refnum<vi>)  [unwired: 1 in, 1 out]
                    n164 = call "Set_Cluster_Argument.vi"("Clust Refnum"=w206, "Argument List In"=w210) -> ("Argument List Out"=w209:string[])  [unwired: 1 in]
                  }
                  n165 = call "Set_Argument.vi"("Enable"=FALSE, "Argument"="API_Init", "Argument List In"=w202) -> ("Argument List Out"=w201:string[])
                }
              }
              n166 = property on="Argument List Out" class="Arr (strict)"("Value"=w195) -> ()  [unwired: 2 in, 2 out]
            }
          }
          n167 = property class="VI"(reference=w85, "Front Panel.Open"=FALSE ("Front Panel Window:Open"), "FP.Behavior"=T3."Default" ("Front Panel Window:Behavior")) -> (reference out=w86:refnum<vi>)  [unwired: 1 in, 1 out]
          n168 = Close Reference(reference=w86) -> ()  [unwired: 1 in, 1 out]
        }
        frame "Start" {
          n169 = property on="prep_time" class="DigNum (strict)"() -> ("Value"=w217:dbl)  [unwired: 2 in, 2 out]
          n170 = Greater Than 0?(x=w217) -> (x > 0?=w216:bool)
          n171 = Not(x=w214) -> (.not. x?=w213:bool)
          n172 = property on="Argument List Out" class="Arr (strict)"() -> ("Value"=w212:string[])  [unwired: 2 in, 2 out]
          n173 = And(x=w213, y=w216) -> (x .and. y?=w215:bool)
          n174 = call "Set_Argument.vi"("Enable"=FALSE, "Argument"="run_started", "Argument List In"=w212) -> ("Argument List Out"=w211:string[])
          n175 = case shown="True" w215 {
            frame False {
            }
            frame True {
              n176 = property on="Ga_bubbler" class="Clust (strict)"() -> ("Value"=w226:T1)  [unwired: 2 in, 2 out]
              n177 = property on="Zn_bubbler" class="Clust (strict)"() -> ("Value"=w220:T1)  [unwired: 2 in, 2 out]
              n178 = property on="Al_bubbler" class="Clust (strict)"() -> ("Value"=w227:T2)  [unwired: 2 in, 2 out]
              n179 = property on="In_bubbler" class="Clust (strict)"() -> ("Value"=w225:T2)  [unwired: 2 in, 2 out]
              n180 = property on="P_gas" class="Clust (strict)"() -> ("Value"=w224:T2)  [unwired: 2 in, 2 out]
              n181 = property on="Se_bubbler" class="Clust (strict)"() -> ("Value"=w221:T1)  [unwired: 2 in, 2 out]
              n182 = property on="As_gas" class="Clust (strict)"() -> ("Value"=w223:T2)  [unwired: 2 in, 2 out]
              n183 = property on="P_bubbler" class="Clust (strict)"() -> ("Value"=w222:T2)  [unwired: 2 in, 2 out]
              n184 = call "Set_V_III.vi"("Se bubbler"=w221, "P bubbler"=w222, "As gas"=w223, "P gas"=w224, "Run Started"=FALSE, "Zn bubbler"=w220, "In bubbler"=w225, "Ga bubbler"=w226, "Al bubbler"=w227) -> ()  [unwired: 3 in]
            }
          }
          n185 = property on="Argument List Out" class="Arr (strict)"("Value"=w211) -> ()  [unwired: 2 in, 2 out]
        }
        frame "Run" {
          n186 = property on="source array" class="Arr (strict)"() -> ("Value"=w229:refnum<vi>[])  [unwired: 2 in, 2 out]
          n187 = stacked-sequence {
            tunnel: w231 -> [_ w236 _ _]
            tunnel: w230 -> [_ _ _ w268]
            tunnel: w229 -> [_ _ w238 _]
            frame #0 {
              n188 = property on="Argument List Out" class="Arr (strict)"() -> ("Value"=w233:string[])  [unwired: 2 in, 2 out]
              n189 = call "Get_Argument.vi"("Argument"="run_started", "Argument List"=w233) -> ("Enabled"=w232:bool)
              n190 = property on="run started" class="Bool (strict)"("Value"=w232) -> ()  [unwired: 2 in, 2 out]
            }
            frame #1 {
              n191 = property on="prep_time" class="DigNum (strict)"() -> ("Value"=w237:dbl)  [unwired: 2 in, 2 out]
              n192 = Greater Or Equal?(x=w236, y=w237) -> (x >= y?=w235:bool)
              n193 = property on="prep_done" class="Bool (strict)"("Value"=w235) -> ()  [unwired: 2 in, 2 out]
            }
            frame #2 {
              n194 = property on="run started" class="Bool (strict)"() -> ("Value"=w239:bool)  [unwired: 2 in, 2 out]
              n195 = Not(x=w239) -> (.not. x?=w241:bool)
              n196 = for {
                shift-right: [w253] -> _
                shift-left: TRUE ("first") -> [w251]
                tunnel: w241 -> [w252]
                tunnel: w238 -> [w245] mode=indexing
                w244 = refnum<vi> refnum  # Cluster
                n197 = To More Specific Class(target class=w244, reference=w245) -> (specific class reference=w243:refnum<vi>)  [unwired: 1 in, 1 out]
                n198 = property class="Clust"(reference=w243) -> ("Controls[]"=w247:refnum<vi>[])  [unwired: 1 in, 2 out]
                n199 = Array Size(array=w247) -> (size(s)=w246:i32)
                n200 = case shown="6" w246 {
                  tunnel: [w260 w263] -> w249
                  tunnel: w243 -> [w260 w261]
                  frame Default {
                  }
                  frame 6 {
                    n201 = control-ref of="Ga bubbler"() -> (w262:refnum<vi>)
                    n202 = To More Specific Class(target class=w262, reference=w261) -> (specific class reference=w266:refnum<vi>)  [unwired: 1 in, 1 out]
                    n203 = property class="Clust (strict)"(reference=w266) -> ("Controls[]"=w265:refnum<vi>[])  [unwired: 1 in, 2 out]
                    n204 = Index Array(array=w265, index=5) -> (element=w263:refnum<vi>)
                  }
                }
                n205 = control-ref of="Al bubbler"() -> (w250:refnum<vi>)
                n206 = To More Specific Class(target class=w250, reference=w249) -> (specific class reference=w248:refnum<vi>)  [unwired: 1 in, 1 out]
                n207 = property class="Clust (strict)"(reference=w248) -> ("Value"=w259:T2)  [unwired: 1 in, 2 out]
                n208 = Unbundle By Name(w259) -> ("Prep"=w258:bool, "Run"=w257:bool, "Active"=w256:bool, "Name"=w242:string)
                n209 = property on="Status Out" class="Str"() -> ("Value"=w255:string)  [unwired: 2 in, 2 out]
                n210 = call "flow_strings.vi"("string in"=w255, "is first in?"=w251, "use source?"=w256, "name"=w242, "run source?"=w257, "prep source?"=w258, "is prep?"=w252) -> ("string out"=w254:string, "is first out?"=w253:bool)
                n211 = property on="Status Out" class="Str"("Value"=w254) -> ()  [unwired: 2 in, 2 out]
              }
            }
            frame #3 {
              n212 = property on="run started" class="Bool (strict)"() -> ("Value"=w270:bool)  [unwired: 2 in, 2 out]
              n213 = Not(x=w270) -> (.not. x?=w269:bool)
              n214 = property on="prep_done" class="Bool (strict)"() -> ("Value"=w271:bool)  [unwired: 2 in, 2 out]
              n215 = And(x=w271, y=w269) -> (x .and. y?=w267:bool)
              n216 = case shown="True" w267 {
                selector: w267 -> [_ w272]
                tunnel: w268 -> [_ w273]
                frame False {
                }
                frame True {
                  n217 = stacked-sequence {
                    tunnel: w273 -> [w275 _]
                    tunnel: w272 -> [w274 _]
                    frame #0 {
                      n218 = case shown="False" w275 {
                        tunnel: w274 -> [w284 _]
                        frame False {
                          n219 = property on="Ga_bubbler" class="Clust (strict)"() -> ("Value"=w282:T1)  [unwired: 2 in, 2 out]
                          n220 = property on="In_bubbler" class="Clust (strict)"() -> ("Value"=w281:T2)  [unwired: 2 in, 2 out]
                          n221 = property on="P_gas" class="Clust (strict)"() -> ("Value"=w280:T2)  [unwired: 2 in, 2 out]
                          n222 = property on="Al_bubbler" class="Clust (strict)"() -> ("Value"=w283:T2)  [unwired: 2 in, 2 out]
                          n223 = property on="Zn_bubbler" class="Clust (strict)"() -> ("Value"=w276:T1)  [unwired: 2 in, 2 out]
                          n224 = property on="Se_bubbler" class="Clust (strict)"() -> ("Value"=w277:T1)  [unwired: 2 in, 2 out]
                          n225 = property on="As_gas" class="Clust (strict)"() -> ("Value"=w279:T2)  [unwired: 2 in, 2 out]
                          n226 = property on="P_bubbler" class="Clust (strict)"() -> ("Value"=w278:T2)  [unwired: 2 in, 2 out]
                          n227 = call "Set_V_III.vi"("Se bubbler"=w277, "P bubbler"=w278, "As gas"=w279, "P gas"=w280, "Run Started"=w284, "Zn bubbler"=w276, "In bubbler"=w281, "Ga bubbler"=w282, "Al bubbler"=w283) -> ()  [unwired: 3 in]
                        }
                        frame True {
                        }
                      }
                    }
                    frame #1 {
                      n228 = property on="Argument List Out" class="Arr (strict)"() -> ("Value"=w285:string[])  [unwired: 2 in, 2 out]
                      n229 = call "Set_Argument.vi"("Enable"=TRUE, "Argument"="run_started", "Argument List In"=w285) -> ("Argument List Out"=w286:string[])
                      n230 = property on="Argument List Out" class="Arr (strict)"("Value"=w286) -> ()  [unwired: 2 in, 2 out]
                    }
                  }
                }
              }
            }
          }
        }
        frame "End" {
        }
        frame "Idle" {
        }
      }
    }
  }
